vi "单步启动选择对话框.vi"() -> (1 "确定":bool, 3 "启动选择 2":u16(ring) items=["进水样", "进蒸馏水", "进标液", "进质控样", "进加标回收样", "进高锰酸钾", "进草酸钠", "进硫酸", "加热", "电磁搅拌", "排液", ""])   [LabVIEW 2016, in "斯坦道CODMn.lvlib"]
panel:
  in  "取消":bool
  in  "启动选择":u16(ring) items=["进水样", "进蒸馏水", "进标液", "进质控样", "进加标回收样", "进高锰酸钾", "进草酸钠", "进硫酸", "加热", "电磁搅拌", "排液"]
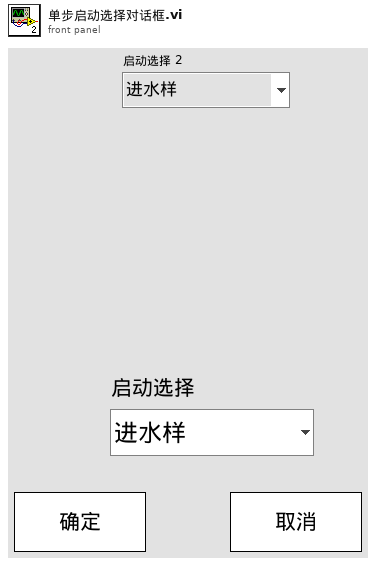
[diagram p1: front panel]
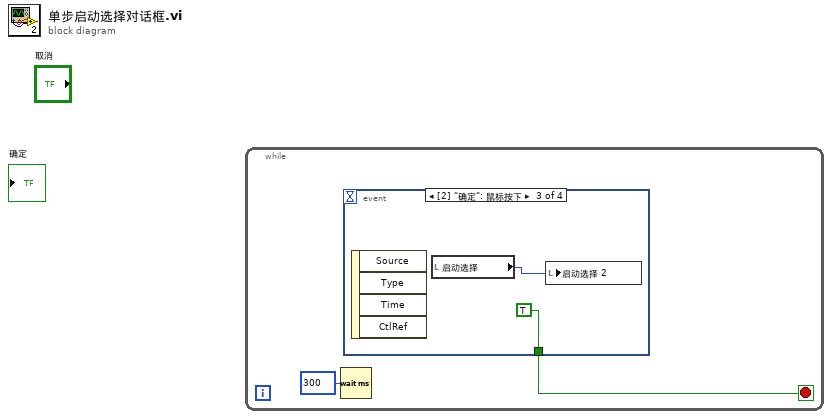
[diagram p0: block diagram]
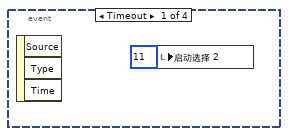
[diagram p2: hidden frame]
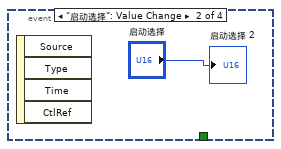
[diagram p3: hidden frame]
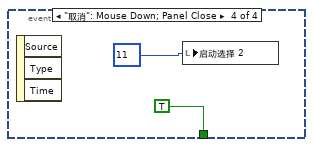
[diagram p4: hidden frame]
diagram:
  n1 = while {
    stop <- w2 stop-if-true
    n2 = Wait (ms)(milliseconds to wait=u32 300 ("等待时间（毫秒）")) -> ()  [unwired: 1 out]
    n3 = event shown="[2] \"确定\": 鼠标按下" {
      selector: _ -> [_ _ _ _]
      dyn-events: _ -> [_ _ _ _]
      timeout: _ -> [_ _ _ _]
      tunnel: [_ _ TRUE TRUE] -> w2
      event Timeout {
        w3 = u16 11 items=["进水样", "进蒸馏水", "进标液", "进质控样", "进加标回收样", "进高锰酸钾", "进草酸钠", "进硫酸", "加热", "电磁搅拌", "排液", ""] ("启动选择 2")
        n4 = event-data() -> ()  [unwired: 1 in, 3 out]
        n5 = local write "启动选择 2"(w3) -> ()
      }
      event "启动选择": Value Change {
        n6 = event-data() -> ()  [unwired: 1 in, 4 out]
        "启动选择 2" <- "启动选择"
      }
      event "确定": Mouse Down {
        n7 = event-data() -> ()  [unwired: 1 in, 4 out]
        n8 = local read "启动选择"() -> (w5:u16)
        n9 = local write "启动选择 2"(w5) -> ()
      }
      event "取消": Mouse Down; Panel Close {
        w7 = u16 11 items=["进水样", "进蒸馏水", "进标液", "进质控样", "进加标回收样", "进高锰酸钾", "进草酸钠", "进硫酸", "加热", "电磁搅拌", "排液", ""] ("启动选择 2")
        n10 = event-data() -> ()  [unwired: 1 in, 3 out]
        n11 = local write "启动选择 2"(w7) -> ()
      }
    }
  }
